vi "G# - DependencyInjectionUsingExternalCreateProcessWithDefaultConstructor.vi"() -> ()   [LabVIEW 2020]
doc: "Dependency Injection with G# External create process run G# Default Constructor\nThis example demonstrates how to use the G#Object_GenericDefaultConstructor.vi\nand G#Object_Open.vi together with the external create process.\n\nBy using the G# Debugger found in Tools->G# Debugger a text log can be followed showing how the objects were created and destroyed. Run the with execution highlighted (lightbulb)."
uses:
  MyG#SubClass_class/MyG#SubClass.lvclass
  vi.lib/addons/_AddQ/G#Object/G#Object.lvclass
panel:
  out "class path":path
  in  "MySubAttribute in":dbl=5.0
  in  "MyAttribute in":dbl=2.0
  in  "error in (no error)":errorcluster
  in  "Use external create process":bool=TRUE
  in  "Run the destructor and garbage collector?":bool=TRUE
  out "MySubAttribute out":dbl
  out "MyAttribute out":dbl
  out "class name":string
  out "error out":errorcluster
  out "OK":bool
  out "# of objects killed":i32
  # "Dependency Injection with G# External create process run G# Default Constructor\nThis example demonstrates how to use the G#Object_GenericDefaultConstructor.vi\nand G#Object_Open.vi together with the external create process.\n\nBy using the G# Debugger found in Tools->G# Debugger a text log can be followed showing how the objects\nwere created and destroyed. Run the with execution highlighted (lightbulb)"
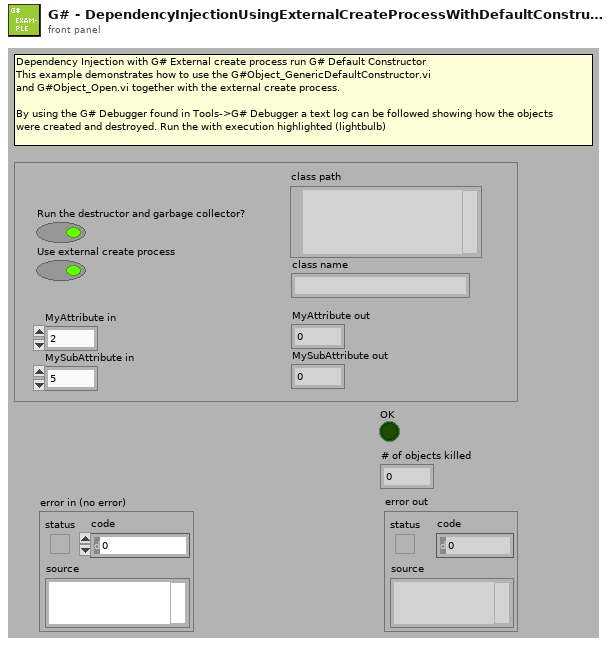
[diagram p1: front panel]
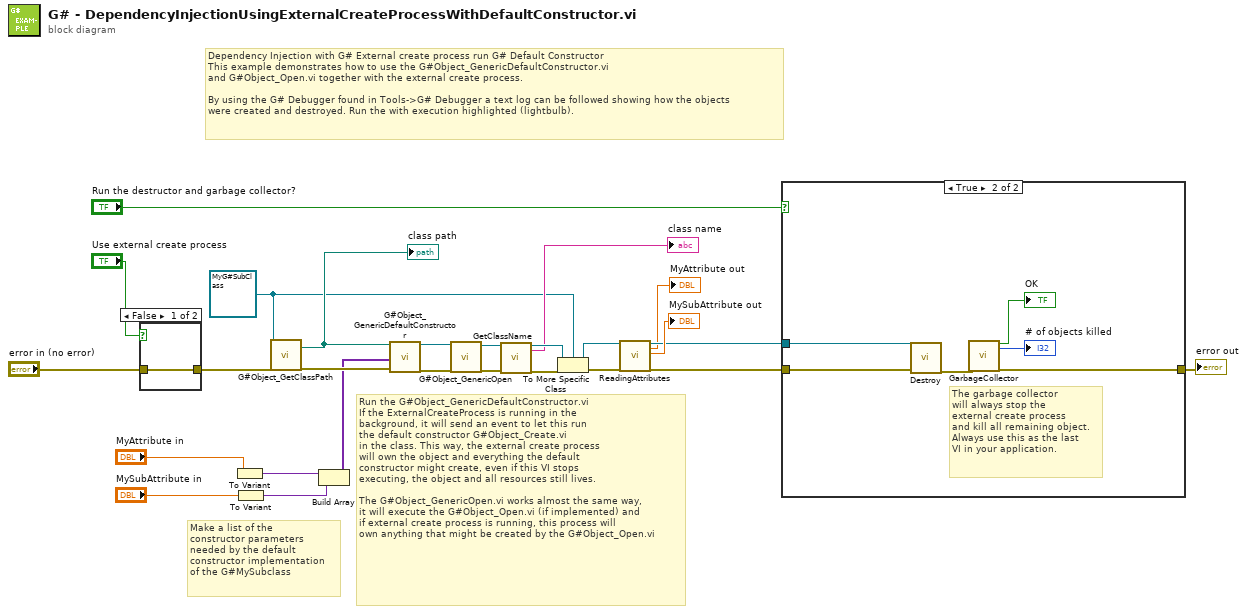
[diagram p0: block diagram]
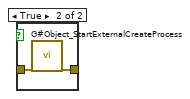
[diagram p2: hidden frame]
diagram:
  w8 = refnum<class "MyG#SubClass.lvclass"> refnum ("MyG#SubClass.lvclass")
  # "Dependency Injection with G# External create process run G# Default Constructor\nThis example demonstrates how to use the G#Object_GenericDefaultConstructor.vi\nand G#Object_Open.vi together with the external create process.\n\nBy using the G# Debugger found in Tools->G# Debugger a text log can be followed showing how the objects\nwere created and destroyed. Run the with execution highlighted (lightbulb)."
  # "Make a list of the \nconstructor parameters\nneeded by the default\nconstructor implementation\nof the G#MySubclass"
  # "Run the G#Object_GenericDefaultConstructor.vi\nIf the ExternalCreateProcess is running in the\nbackground, it will send an event to let this run\nthe default constructor G#Object_Create.vi\nin the class. This way, the external create process\nwill own the object and everything the default\nconstructor might create, even if this VI stops\nexecuting, the object and all resources still lives.\n\nThe G#Object_GenericOpen.vi works almost the same way,\nit will execute the G#Object_Open.vi (if implemented) and\nif external create process is running, this process will\nown anything that might be created by the G#Object_Open.vi"
  n1 = case shown="False" "Use external create process" {
    tunnel: [w27 w29] -> w26
    tunnel: "error in (no error)" -> [w27 w28]
    frame False {
    }
    frame True {
      n2 = call "G#Object_StartExternalCreateProcess.vi"("error in (no error)"=w28) -> ("error out"=w29:errorcluster)  [unwired: 18 in]
    }
  }
  n3 = To Variant(anything="MyAttribute in") -> (Variant=w22:variant)
  n4 = To Variant(anything="MySubAttribute in") -> (Variant=w21:variant)
  n5 = call-dynamic "G#Object_GetClassPath.vi"("reference in"=w8, "error in (no error)"=w26) -> ("class path"=w24:path, "error out"=w25:errorcluster)  [unwired: 15 in, 1 out]
  "class path" <- w24
  n6 = Build Array(w22, w21) -> (w18:variant[])
  n7 = call "G#Object_GenericDefaultConstructor.vi"("class path"=w24, "control values"=w18, "error in (no error)"=w25) -> ("reference out"=w4:refnum<class "G#Object.lvclass">, "error out"=w3:errorcluster)  [unwired: 14 in, 1 out]
  n8 = call-dynamic "G#Object_GenericOpen.vi"("reference in"=w4, "error in (no error)"=w3) -> ("reference out"=w1:refnum<class "G#Object.lvclass">, "error out"=w2:errorcluster)  [unwired: 15 in, 1 out]
  n9 = call-dynamic "GetClassName.vi"("reference in"=w1, "error in (no error)"=w2) -> ("reference out"=w15:refnum<class "G#Object.lvclass">, "class name"=→"class name":string, "error out"=w16:errorcluster)  [unwired: 13 in, 2 out]
  n10 = To More Specific Class(target class=w8, reference=w15, error in=w16) -> (specific class reference=w13:refnum<class "MyG#SubClass.lvclass">, error out=w14:errorcluster)
  n11 = call-dynamic "ReadingAttributes.vi"("reference in"=w13, "error in (no error)"=w14) -> ("reference out"=w10:refnum<class "MyG#SubClass.lvclass">, "MyAttribute"=→"MyAttribute out":dbl, "MySubAttribute"=→"MySubAttribute out":dbl, "error out"=w12:errorcluster)  [unwired: 14 in]
  n12 = case shown="True" "Run the destructor and garbage collector?" {
    tunnel: [w30 w34] -> w17
    tunnel: w12 -> [w30 w33]
    tunnel: w10 -> [_ w32]
    frame False {
      # "If this case is executed,if  the external create process is running\nit will not be stopped and objects continue to live. If the\nexternal create process is not running, LabVIEW will automatically\ngarbage collect and kill and queue etc.\n\nOpen the G#Debugger before running this example\nto verify that objects still lives if external create process is running.\nKill the objects and external create process that manually\ntrigger Garbage collector in the G#Debugger."
    }
    frame True {
      # "The garbage collector\nwill always stop the\nexternal create process\nand kill all remaining object.\nAlways use this as the last\nVI in your application."
      n13 = call-dynamic "Destroy.vi"("reference in"=w32, "error in (no error)"=w33) -> ("error out"=w35:errorcluster)  [unwired: 16 in, 1 out]
      n14 = call "GarbageCollector.vi"("error in (no error)"=w35) -> ("OK"=→"OK":bool, "# of objects killed"=→"# of objects killed":i32, "error out"=w34:errorcluster)  [unwired: 16 in]
    }
  }
  "error out" <- w17
